vi "XIPIN_DUC_DDC_Compiler_3_0.vi"   [LabVIEW 2017]
doc: "Digital Up/Down Converters (DUC/DDC) are important components in the signal processing chains of many digital communications systems. The Xilinx DUC/DDC Compiler LogiCORE provides users with means to rapidly implement these functions for a range of wireless interface standards based on system-level parameters. The core implementation is delivered through the Xilinx Vivado IP Catalog, and is designed to take advantage of the advanced features of Xilinx FPGA devices.\n------------------------------------\n<b>Need License</b> : No\n<b>Interface</b> : AXI4-Stream"
uses:
  <vilib>/rvi/XilinxIP/XIPIN_XNode/niFpgaXIPIN.xnode
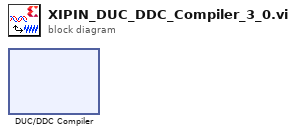
[diagram p0: block diagram]
diagram:
  n1 = xnode ("DUC/DDC Compiler")() -> ()
